vi "CLI_Disable Source Separation.vi"(11 "CLI Arguments":string[](array[string])) -> (2 "Output":string, 3 "Error Code":i32)   [LabVIEW 2014]
doc: "Copyright (c) 2018 Sze Howe Koh\n\nThis Source Code Form is subject to the terms of the Mozilla Public License, v. 2.0. If a copy of the MPL was not distributed with this file, You can obtain one at http://mozilla.org/MPL/2.0/."
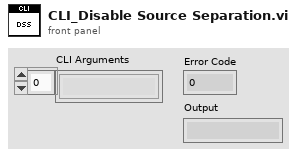
[diagram p1: front panel]
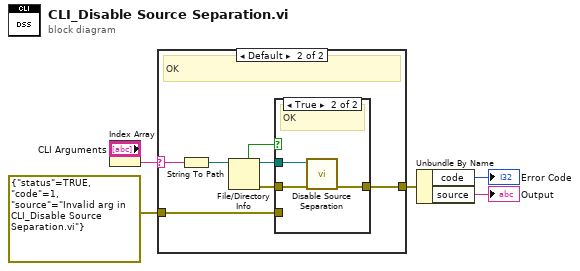
[diagram p0: block diagram]
diagram:
  n1 = Index Array(array="CLI Arguments") -> (element=w5:string)  [unwired: 1 in]
  n2 = case shown="Default" w5 {
    selector: w5 -> [_ w14]
    tunnel: [w7 w9] -> w4
    tunnel: errorcluster {"status"=TRUE, "code"=1, "source"="Invalid arg in CLI_Disable Source Separation.vi"} -> [w7 w8]
    frame "" {
      # "Empty string -> System root directory\nDON'T RUN!!!"
    }
    frame Default {
      # "OK"
      n3 = String To Path(string=w14) -> (path=w13:path)
      n4 = File/Directory Info(path=w13) -> (path out=w11:path, directory=w10:bool, error out=w12:errorcluster)  [unwired: 1 in, 4 out]
      n5 = case shown="True" w10 {
        tunnel: w12 -> [_ w18]
        tunnel: w11 -> [_ w17]
        tunnel: [w15 w16] -> w9
        tunnel: w8 -> [w15 _]
        frame False {
          # "Not a folder"
        }
        frame True {
          # "OK"
          n6 = call "Disable Source Separation.vi"("Error In"=w18, "Root Path"=w17) -> ("Error Out"=w16:errorcluster)  [unwired: 9 in]
        }
      }
    }
  }
  n7 = Unbundle By Name(w4) -> ("code"=→"Error Code":i32, "source"=→"Output":string)
